vi "WriteDigioBits2_DAQmx.vi"(8 "error in":errorcluster, 9 "Bits to write":T1, 10 "Number":u32, 11 "DO Task":refnum<k21>="BlueSimple_DO") -> (0 "error out":errorcluster)   [LabVIEW 2010]
uses:
  Controls/Bits to Write.ctl
  <vilib>/DAQmx/write.llb/DAQmx Write (Digital 1D Bool NChan 1Samp 1Line).vi
  <vilib>/daqmx/miscellaneous.llb/DAQmx Fill In Error Info.vi
panel:
  in  "line mask":i32=-65536 format="%b"
  in  "pattern":u32 format="%b"
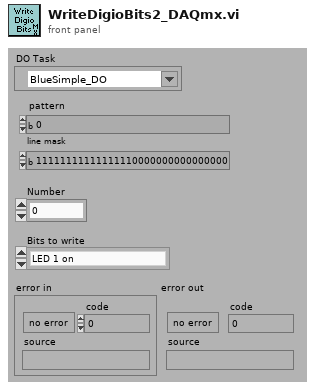
[diagram p1: front panel]
types:
  T1 = typedef "Bits to Write.ctl" = enum16{"LED 1 on", "LED 1 off", "LED 2 on", "LED 2 off", "LED 3 on", "LED 3 off", "LED 4 on", "LED 4 off", "All LEDs on", "All LEDs off", "In trial on", "In trial off", "Buzzer on", "Buzzer off", "Reward on", "Reward off", "Target number", "Trial type preQ on", "Trial type preQ off", "Error on", "Error off", "Trial number", "DBS on", "DBS off", "Sine on", "Sine off", "All Bits On", "All Bits Off", "Init", "Specify mask/pattern"}
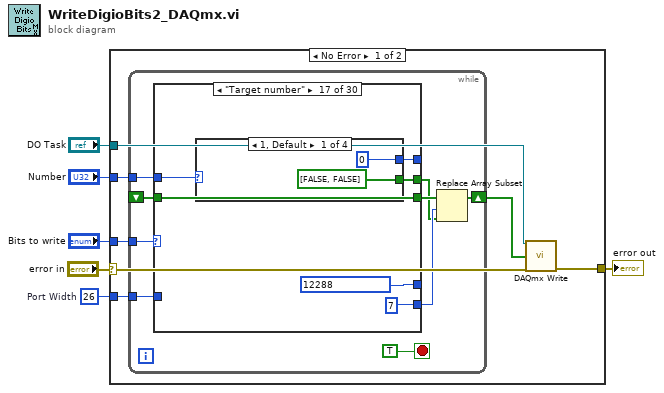
[diagram p0: block diagram]
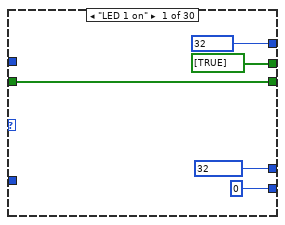
[diagram p2: hidden frame]
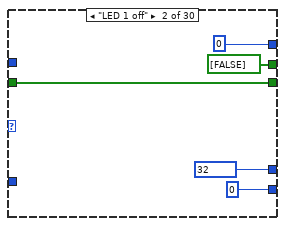
[diagram p3: hidden frame]
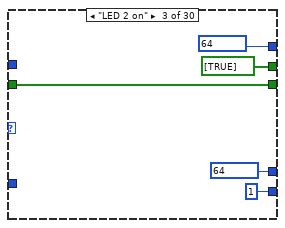
[diagram p4: hidden frame]
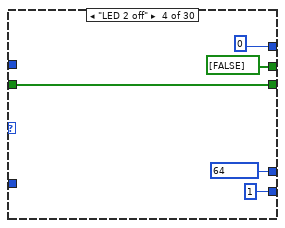
[diagram p5: hidden frame]
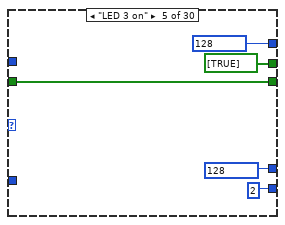
[diagram p6: hidden frame]
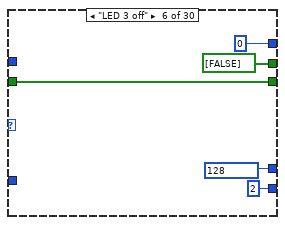
[diagram p7: hidden frame]
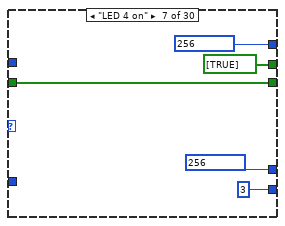
[diagram p8: hidden frame]
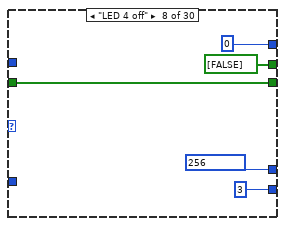
[diagram p9: hidden frame]
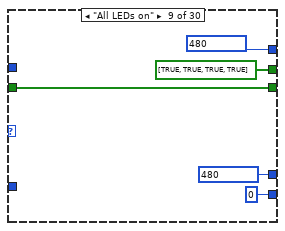
[diagram p10: hidden frame]
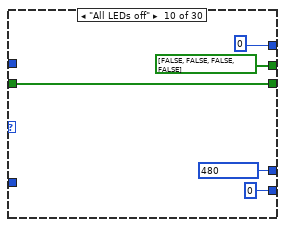
[diagram p11: hidden frame]
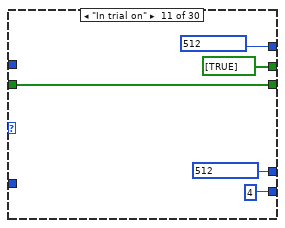
[diagram p12: hidden frame]
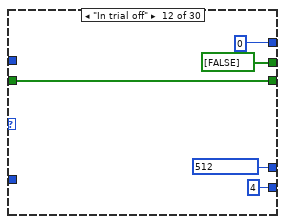
[diagram p13: hidden frame]
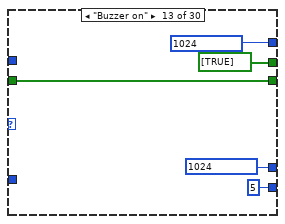
[diagram p14: hidden frame]
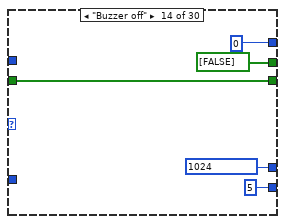
[diagram p15: hidden frame]
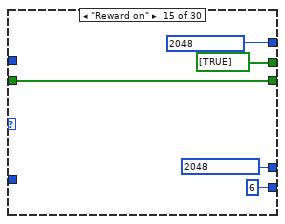
[diagram p16: hidden frame]
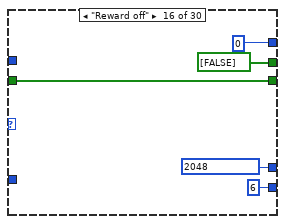
[diagram p17: hidden frame]
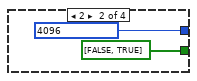
[diagram p18: hidden frame]
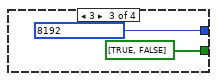
[diagram p19: hidden frame]
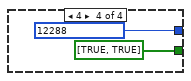
[diagram p20: hidden frame]
diagram:
  w2 = 26  # Port Width
  n1 = case shown="No Error" "error in" {
    selector: "error in" -> [w8 w183]
    tunnel: "Bits to write" -> [w13 _]
    tunnel: "Number" -> [w12 _]
    tunnel: [w11 w183] -> w4
    tunnel: "DO Task" -> [w10 _]
    tunnel: w2 -> [w9 _]
    frame No Error {
      n2 = while {
        tunnel: w13 -> [w22]
        tunnel: w12 -> [w21]
        tunnel: w9 -> [w20]
        shift-right: [w17] -> w7
        shift-left: _ -> [w19]
        stop <- TRUE stop-if-true
        n3 = case shown="\"Target number\"" w22 {
          tunnel: [u32 32 ("line mask") u32 0 ("line mask") u32 64 ("line mask") u32 0 ("line mask") u32 128 ("line mask") u32 0 ("line mask") u32 256 ("line mask") u32 0 ("line mask") u32 480 ("line mask") u32 0 ("line mask") u32 512 ("line mask") u32 0 ("line mask") u32 1024 ("line mask") u32 0 ("line mask") u32 2048 ("line mask") u32 0 ("line mask") w106 u32 16384 ("line mask") u32 0 ("line mask") u32 32768 ("line mask") u32 0 ("line mask") _ u32 268435456 ("line mask") u32 0 ("line mask") u32 536870912 ("line mask") u32 0 ("line mask") _ _ _ _] -> _
          tunnel: [32 ("line mask") 32 ("line mask") 64 ("line mask") 64 ("line mask") 128 ("line mask") 128 ("line mask") 256 ("line mask") 256 ("line mask") 480 ("line mask") 480 ("line mask") 512 ("line mask") 512 ("line mask") 1024 ("line mask") 1024 ("line mask") 2048 ("line mask") 2048 ("line mask") 12288 ("line mask") 16384 ("line mask") 16384 ("line mask") 32768 ("line mask") 32768 ("line mask") 268369920 ("line mask") 268435456 ("line mask") 268435456 ("line mask") 536870912 ("line mask") 536870912 ("line mask") _ _ _ _] -> _
          tunnel: w21 -> [_ _ _ _ _ _ _ _ _ _ _ _ _ _ _ _ w107 _ _ _ _ w142 _ _ _ _ _ _ _ _]
          tunnel: w20 -> [_ _ _ _ _ _ _ _ _ _ _ _ _ _ _ _ _ _ _ _ _ _ _ _ _ _ w167 w172 w178 _]
          tunnel: [w24 w29 w34 w39 w44 w49 w54 w59 w64 w69 w74 w79 w84 w89 w94 w99 w104 w118 w123 w128 w133 w144 w147 w152 w157 w162 w170 w175 w177 w182] -> w18
          tunnel: w19 -> [w24 w29 w34 w39 w44 w49 w54 w59 w64 w69 w74 w79 w84 w89 w94 w99 w104 w118 w123 w128 w133 w144 w147 w152 w157 w162 w170 w175 _ w182]
          tunnel: [0 ("line mask") 0 ("line mask") 1 ("line mask") 1 ("line mask") 2 ("line mask") 2 ("line mask") 3 ("line mask") 3 ("line mask") 0 ("line mask") 0 ("line mask") 4 ("line mask") 4 ("line mask") 5 ("line mask") 5 ("line mask") 6 ("line mask") 6 ("line mask") 7 ("line mask") 9 ("line mask") 9 ("line mask") 10 ("line mask") 10 ("line mask") 11 ("line mask") 23 ("line mask") 23 ("line mask") 24 ("line mask") 24 ("line mask") 0 ("line mask") 0 ("line mask") 0 ("line mask") 0 ("line mask")] -> w15
          tunnel: [bool[] [TRUE] bool[] [FALSE] bool[] [TRUE] bool[] [FALSE] bool[] [TRUE] bool[] [FALSE] bool[] [TRUE] bool[] [FALSE] bool[] [TRUE, TRUE, TRUE, TRUE] bool[] [FALSE, FALSE, FALSE, FALSE] bool[] [TRUE] bool[] [FALSE] bool[] [TRUE] bool[] [FALSE] bool[] [TRUE] bool[] [FALSE] w105 bool[] [TRUE] bool[] [FALSE] bool[] [TRUE] bool[] [FALSE] w137 bool[] [TRUE] bool[] [FALSE] bool[] [TRUE] bool[] [FALSE] w166 w171 w177 bool[] [FALSE]] -> w14
          frame "LED 1 on" {
          }
          frame "LED 1 off" {
          }
          frame "LED 2 on" {
          }
          frame "LED 2 off" {
          }
          frame "LED 3 on" {
          }
          frame "LED 3 off" {
          }
          frame "LED 4 on" {
          }
          frame "LED 4 off" {
          }
          frame "All LEDs on" {
          }
          frame "All LEDs off" {
          }
          frame "In trial on" {
          }
          frame "In trial off" {
          }
          frame "Buzzer on" {
          }
          frame "Buzzer off" {
          }
          frame "Reward on" {
          }
          frame "Reward off" {
          }
          frame "Target number" {
            n4 = case shown="1, Default" w107 {
              tunnel: [u32 0 ("line mask") u32 4096 ("line mask") u32 8192 ("line mask") u32 12288 ("line mask")] -> w106
              tunnel: [bool[] [FALSE, FALSE] bool[] [FALSE, TRUE] bool[] [TRUE, FALSE] bool[] [TRUE, TRUE]] -> w105
              frame 1, Default {
              }
              frame 2 {
              }
              frame 3 {
              }
              frame 4 {
              }
            }
          }
          frame "Trial type preQ on" {
          }
          frame "Trial type preQ off" {
          }
          frame "Error on" {
          }
          frame "Error off" {
          }
          frame "Trial number" {
            n5 = Number To Boolean Array(number=w142) -> (Boolean array=w138:bool[])
            n6 = Initialize Array(TRUE, 12 ("length")) -> (w139:bool[])
            n7 = And(x=w138, y=w139) -> (x .and. y?=w137:bool[])
          }
          frame "DBS on" {
          }
          frame "DBS off" {
          }
          frame "Sine on" {
          }
          frame "Sine off" {
          }
          frame "All Bits Off" {
            n8 = Initialize Array(FALSE, w167) -> (w166:bool[])
          }
          frame "All Bits On" {
            n9 = Initialize Array(TRUE, w172) -> (w171:bool[])
          }
          frame "Init", Default {
            n10 = Initialize Array(FALSE, w178) -> (w177:bool[])
          }
          frame "Specify mask/pattern" {
            # "This Needs to be Added!"
          }
        }
        n11 = Replace Array Subset(array=w18, new element=w14, index=w15) -> (w17:bool[])
      }
      n12 = call-poly <vilib>:"DAQmx Write.vi"("task/channels in"=w10, "data"=w7, "error in"=w8) -> ("error out"=w11:errorcluster)  [unwired: 10 in, 2 out]
    }
    frame Error {
    }
  }
  "error out" <- w4
